vi "PixyCam_SetLED.vi"(0 "PixyCamDevRef":T1, 5 "Red":u8, 7 "Green":u8, 9 "Blue":u8, 11 "error in (no error)":errorcluster) -> (4 "PixyCamDevRef Out":T1, 15 "error out":errorcluster)   [LabVIEW 2016, in "PixyCam_LabVIEW.lvlib"]
uses:
  PixyCam_LabVIEW.lvlib
  Private/PixyCam_DevRef.ctl
  Private/PixyCam_SPI_DevRef.ctl
  <vilib>/Rock Robotics/WPI/SPI/WPI_SPIDevRef.ctl
  <vilib>/Rock Robotics/SystemInterfaces/spilib/spi_bus.ctl
  Private/PixyCam_CommMode.ctl
  Private/PixyCam_SerialByteConstants.ctl
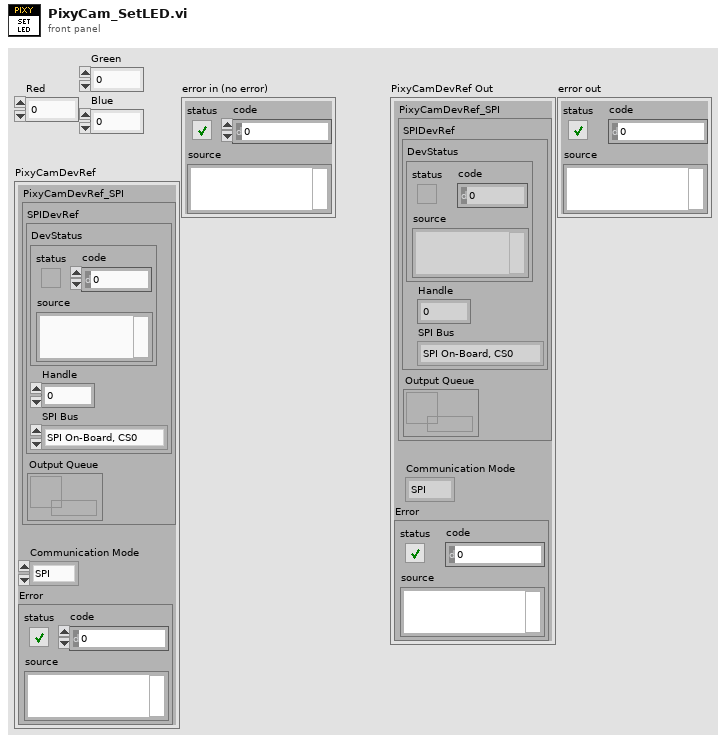
[diagram p1: front panel]
types:
  T1 = typedef "PixyCam_LabVIEW.lvlib/PixyCam_DevRef.ctl" = cluster{"PixyCamDevRef_SPI":T2, "Communication Mode":T5, "Error":errorcluster}
  T2 = typedef "PixyCam_LabVIEW.lvlib/PixyCam_SPI_DevRef.ctl" = cluster{"SPIDevRef":T3, "Output Queue":refnum<queue>}
  T3 = typedef "WPI_SPIDevRef.ctl" = cluster{"DevStatus":errorcluster, "Handle":i32, "SPI Bus":T4}
  T4 = typedef "spi_bus.ctl" = enum16{"SPI On-Board, CS0", "SPI On-Board, CS1", "SPI On-Board, CS2", "SPI On-Board, CS3", "SPI MXP", "Invalid"}
  T5 = typedef "PixyCam_LabVIEW.lvlib/PixyCam_CommMode.ctl" = enum16{"SPI", "I2C", "UART", "Analog", "Digital"}
  T6 = typedef "PixyCam_LabVIEW.lvlib/PixyCam_SerialByteConstants.ctl" = u8
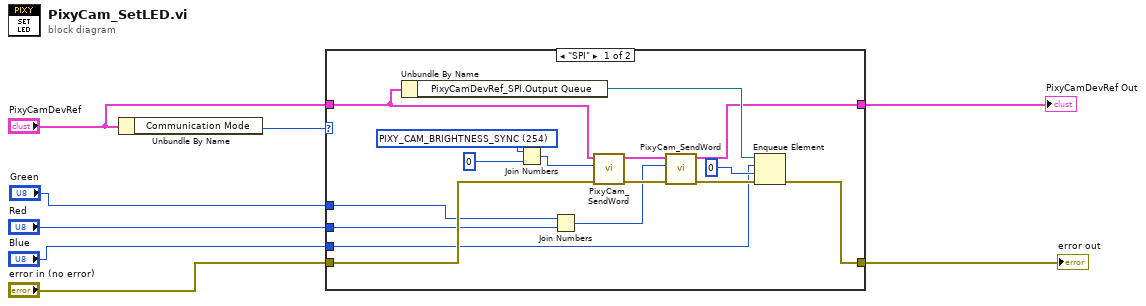
[diagram p0: block diagram]
diagram:
  n1 = Unbundle By Name("PixyCamDevRef") -> ("Communication Mode"=w8:T5)
  n2 = case shown="\"SPI\"" w8 {
    tunnel: "PixyCamDevRef" -> [w20 w26]
    tunnel: "error in (no error)" -> [w24 w25]
    tunnel: "Red" -> [w10 _]
    tunnel: [w15 w26] -> w4
    tunnel: [w17 w25] -> w3
    tunnel: "Green" -> [w11 _]
    tunnel: "Blue" -> [w9 _]
    frame "SPI" {
      w23 = T6 254 items=["PIXY_SYNC_BYTE"=90, "PIXY_SYNC_BYTE_DATA"=91, "PIXY_SERVO_SYNC"=255, "PIXY_CAM_BRIGHTNESS_SYNC"=254, "PIXY_CAM_LED_SYNC"=253] ("SyncByte")
      n3 = Unbundle By Name(w20) -> ("PixyCamDevRef_SPI.Output Queue"=w19:refnum<queue>)
      n4 = Join Numbers(hi=w23, lo=u8 0 ("timeout in ms (-1)")) -> ((hi.lo)=w21:u16)
      n5 = Join Numbers(hi=w11, lo=w10) -> ((hi.lo)=w12:u16)
      n6 = call "PixyCam_SendWord.vi"("error in"=w24, "WriteWord"=w21, "PixyCamDevRef"=w20) -> ("error out"=w14:errorcluster, "PixyCamDevRef Out"=w16:T1)  [unwired: 3 in]
      n7 = call "PixyCam_SendWord.vi"("error in"=w14, "WriteWord"=w12, "PixyCamDevRef"=w16) -> ("error out"=w13:errorcluster, "PixyCamDevRef Out"=w15:T1)  [unwired: 3 in]
      n8 = Enqueue Element(queue=w19, element=w9, timeout in ms (-1)=0, error in (no error)=w13) -> (error out=w17:errorcluster)  [unwired: 2 out]
    }
    frame Default {
    }
  }
  "PixyCamDevRef Out" <- w4
  "error out" <- w3
